vi "DAQ Loop.vi"(8 "error in":errorcluster, 10 "Queues":T1, 11 "Notifiers":T2) -> (0 "error out":errorcluster)   [LabVIEW 2015, in "DAQ.lvlib"]
uses:
  DAQ.lvlib
  support/Message Queue/Message Queue.lvlib
  TypeDefs/DAQ data.ctl
  <vilib>/ErrorRing/Error Ring.xnode
  PLC/PLC.lvlib
  support/Global names.vi
  <vilib>/Utility/error.llb/Error Cluster From Error Code.vi
  support/Message Queue/Message Cluster.ctl
  support/Notifiers/Notifiers.ctl
  support/Notifiers/Notifiers.lvlib
  support/Message Queue/All Message Queues.ctl
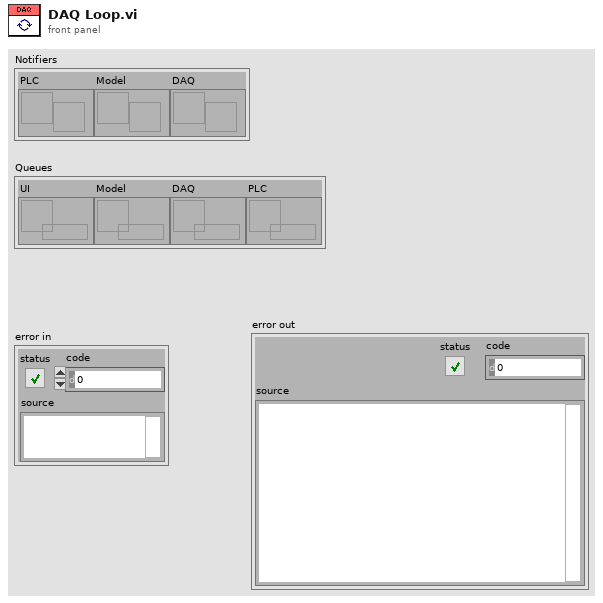
[diagram p1: front panel]
types:
  T1 = typedef "Message Queue.lvlib/All Message Queues.ctl" = cluster{"UI":refnum<queue>, "Model":refnum<queue>, "DAQ":refnum<queue>, "PLC":refnum<queue>}
  T2 = typedef "Notifiers.lvlib/Notifiers.ctl" = cluster{"PLC":refnum<notifier>, "Model":refnum<notifier>, "DAQ":refnum<notifier>}
  T3 = typedef "DAQ.lvlib/DAQ data.ctl" = cluster{"Power switch (DI)":cluster{"Channel":tag, "Data":bool}, "Dispose barrel (DI)":cluster{"Channel":tag, "Data":bool}, "Pump status (DO)":cluster{"Channel":tag, "Data":bool}, "Barrel position (AI)":cluster{"Channel":tag, "Data":dbl}}
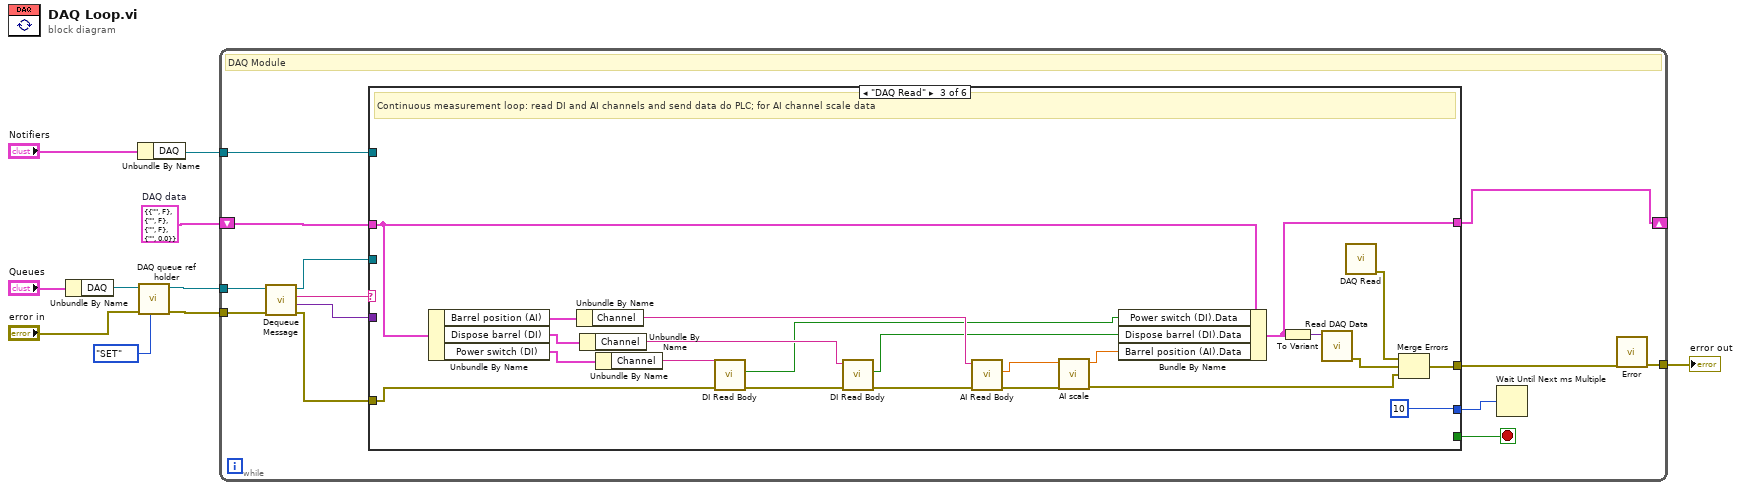
[diagram p0: block diagram]
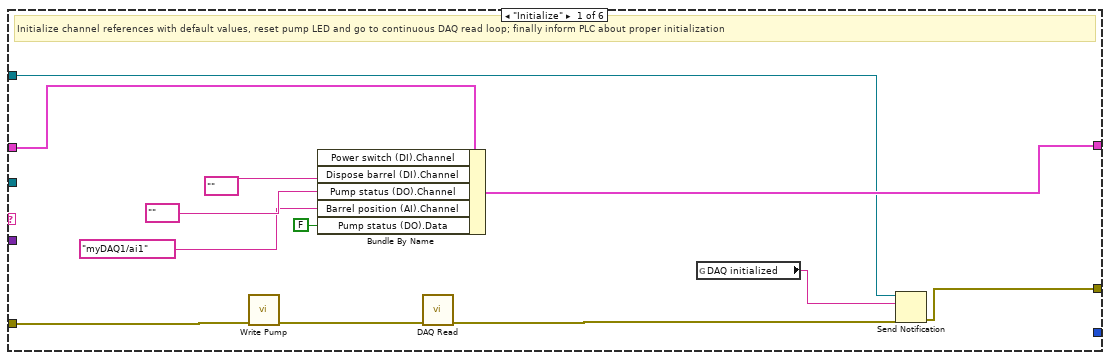
[diagram p2: hidden frame]
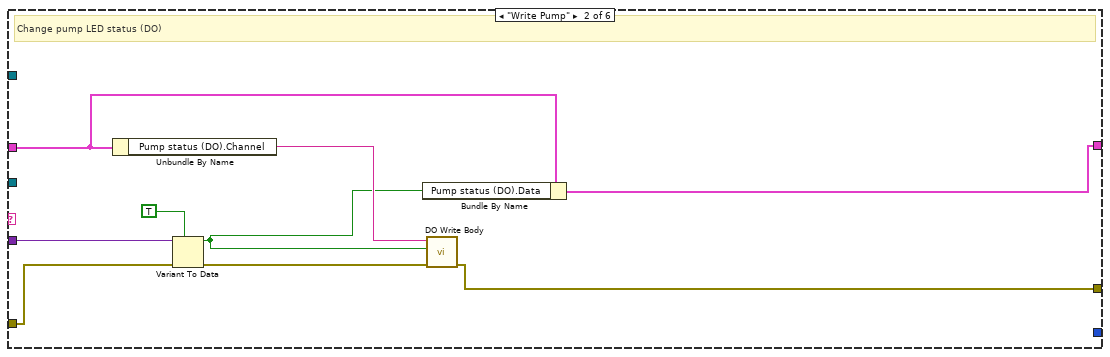
[diagram p3: hidden frame]
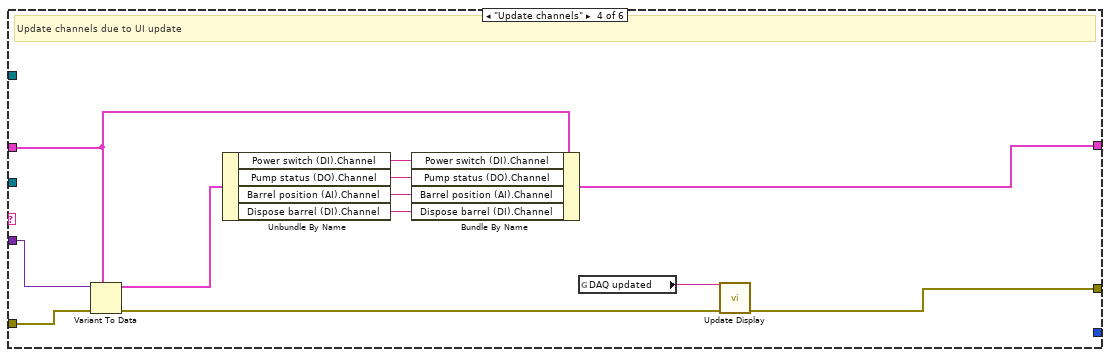
[diagram p4: hidden frame]
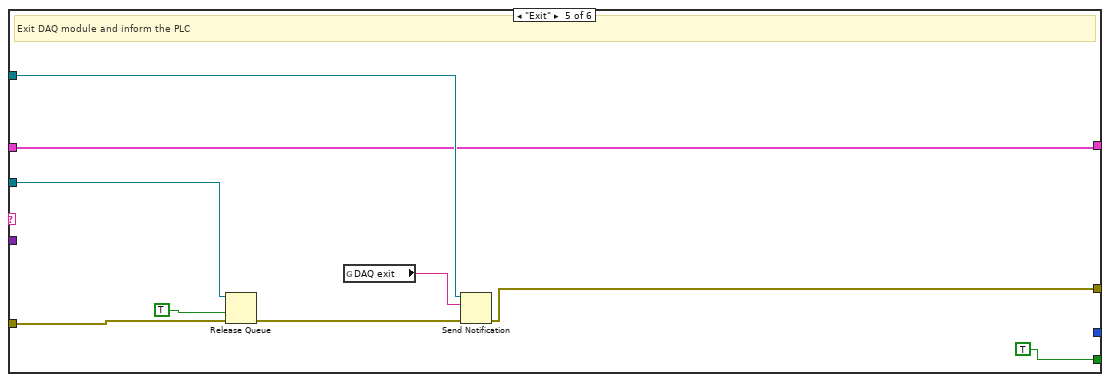
[diagram p5: hidden frame]
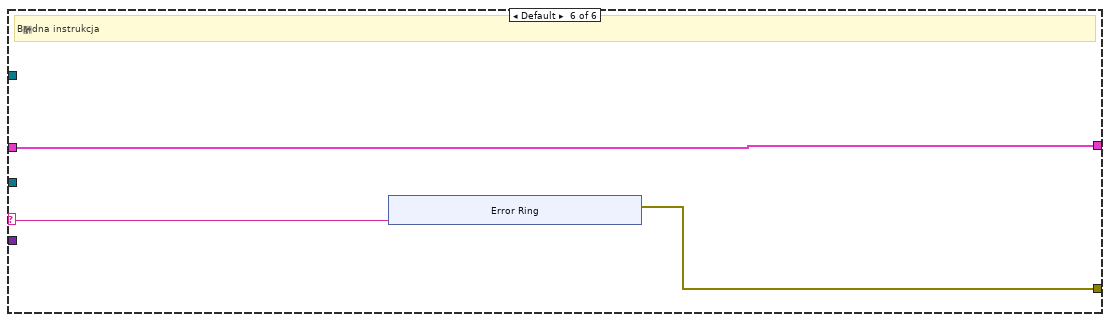
[diagram p6: hidden frame]
diagram:
  w10 = T3 {"Power switch (DI)"={"Channel"="", "Data"=FALSE}, "Dispose barrel (DI)"={"Channel"="", "Data"=FALSE}, "Pump status (DO)"={"Channel"="", "Data"=FALSE}, "Barrel position (AI)"={"Channel"="", "Data"=0.0}}  # DAQ data
  n1 = Unbundle By Name("Queues") -> ("DAQ"=w5:refnum<queue>)
  n2 = Unbundle By Name("Notifiers") -> ("DAQ"=w6:refnum<notifier>)
  n3 = call "DAQ queue ref holder.vi"("Action"=enum16{"GET", "SET"}."SET", "error in"="error in", "Message Queue In"=w5) -> ("error out"=w3:errorcluster, "Input Message Queue"=w4:refnum<queue>)  [unwired: 7 in]
  n4 = while {
    tunnel: w3 -> [w23]
    tunnel: w4 -> [w11]
    tunnel: w6 -> [w19]
    shift-right: [w18] -> _
    shift-left: w10 -> [w16]
    tunnel: [w14] -> w8
    stop <- w20 stop-if-true
    # "DAQ Module"
    n5 = call "Dequeue Message.vi"("error in (no error)"=w23, "Message Queue"=w11) -> ("error out"=w22:errorcluster, "Message Data"=w21:variant, "Message"=w12:string, "dup Message Queue"=w13:refnum<queue>)  [unwired: 6 in]
    n6 = case shown="\"DAQ Read\"" w12 {
      selector: w12 -> [_ _ _ _ _ w89]
      tunnel: w22 -> [w32 w44 w59 w77 w81 _]
      tunnel: [w35 w36 w57 w69 w80 w88] -> w15
      tunnel: w21 -> [_ w43 _ w78 _ _]
      tunnel: [_ _ _ _ TRUE _] -> w20
      tunnel: w13 -> [_ _ _ _ w87 _]
      tunnel: w19 -> [w30 _ _ _ w86 _]
      tunnel: w16 -> [w34 w40 w64 w76 w82 w90]
      tunnel: [w33 w42 w61 w71 w82 w90] -> w18
      tunnel: [_ _ u32 10 ("millisecond multiple") _ _ _] -> w17
      frame "Initialize" {
        # "Initialize channel references with default values, reset pump LED and go to continuous DAQ read loop; finally inform PLC about proper initialization"
        n7 = call "Write Pump.vi"("error in"=w32) -> ("error out"=w31:errorcluster)  [unwired: 10 in]
        n8 = Bundle By Name(cluster=w34, "Dispose barrel (DI).Channel"=tag "", "Pump status (DO).Channel"=tag "", "Barrel position (AI).Channel"=tag "myDAQ1/ai1", "Pump status (DO).Data"=FALSE) -> (w33:T3)  [unwired: 1 in]
        n9 = call "DAQ Read.vi"("error in"=w31) -> ("error out"=w29:errorcluster)  [unwired: 10 in]
        n10 = global read "Global names.vi" "DAQ initialized"() -> (w28:string)
        n11 = Send Notification(notification=w28, notifier=w30, error in (no error)=w29) -> (error out=w35:errorcluster)  [unwired: 1 out]
      }
      frame "Write Pump" {
        # "Change pump LED status (DO)"
        n12 = Unbundle By Name(w40) -> ("Pump status (DO).Channel"=w41:tag)
        n13 = Variant To Data(error in=w44, type=TRUE, Variant=w43) -> (data=w38:bool, error out=w37:errorcluster)
        n14 = Bundle By Name(cluster=w40, "Pump status (DO).Data"=w38) -> (w42:T3)
        n15 = call "DO Write Body.vi"("error in"=w37, "data"=w38, "Channel"=w41) -> ("error out"=w36:errorcluster)  [unwired: 6 in]
      }
      frame "DAQ Read" {
        # "Continuous measurement loop: read DI and AI channels and send data do PLC; for AI channel scale data"
        n16 = Unbundle By Name(w64) -> ("Barrel position (AI)"=w53:cluster{"Channel":tag, "Data":dbl}, "Dispose barrel (DI)"=w51:cluster{"Channel":tag, "Data":bool}, "Power switch (DI)"=w49:cluster{"Channel":tag, "Data":bool})
        n17 = Unbundle By Name(w53) -> ("Channel"=w52:tag)
        n18 = Unbundle By Name(w51) -> ("Channel"=w50:tag)
        n19 = Unbundle By Name(w49) -> ("Channel"=w48:tag)
        n20 = call "DI Read Body.vi"("error in"=w59, "Channel"=w48) -> ("error out"=w66:errorcluster, "data"=w47:bool)  [unwired: 6 in]
        n21 = call "DI Read Body.vi"("error in"=w66, "Channel"=w50) -> ("error out"=w65:errorcluster, "data"=w46:bool)  [unwired: 6 in]
        n22 = call "AI Read Body.vi"("error in"=w65, "Channel"=w52) -> ("error out"=w58:errorcluster, "data"=w54:dbl)  [unwired: 6 in]
        n23 = call "AI scale.vi"("error in"=w58, "Data in"=w54) -> ("error out"=w55:errorcluster, "Data out"=w63:dbl)  [unwired: 8 in]
        n24 = Bundle By Name(cluster=w64, "Power switch (DI).Data"=w47, "Dispose barrel (DI).Data"=w46, "Barrel position (AI).Data"=w63) -> (w61:T3)
        n25 = To Variant(anything=w61) -> (Variant=w60:variant)
        n26 = call "Read DAQ Data.vi"("Message Data"=w60) -> ("error out"=w56:errorcluster)  [unwired: 10 in]
        n27 = call "DAQ Read.vi"() -> ("error out"=w45:errorcluster)  [unwired: 11 in]
        n28 = Merge Errors(w45, w56, w55) -> (w57:errorcluster)
      }
      frame "Update channels" {
        # "Update channels due to UI update"
        n29 = Variant To Data(error in=w77, type=w76, Variant=w78) -> (data=w68:T3, error out=w70:errorcluster)
        n30 = Unbundle By Name(w68) -> ("Power switch (DI).Channel"=w75:tag, "Pump status (DO).Channel"=w74:tag, "Barrel position (AI).Channel"=w73:tag, "Dispose barrel (DI).Channel"=w72:tag)
        n31 = Bundle By Name(cluster=w76, "Power switch (DI).Channel"=w75, "Pump status (DO).Channel"=w74, "Barrel position (AI).Channel"=w73, "Dispose barrel (DI).Channel"=w72) -> (w71:T3)
        n32 = global read "Global names.vi" "DAQ updated"() -> (w67:string)
        n33 = call "Update Display.vi"("error in"=w70, "Message string"=w67) -> ("error out"=w69:errorcluster)  [unwired: 9 in]
      }
      frame "Exit" {
        # "Exit DAQ module and inform the PLC"
        n34 = Release Queue(queue=w87, force destroy? (F)=TRUE, error in (no error)=w81) -> (error out=w85:errorcluster)  [unwired: 2 out]
        n35 = global read "Global names.vi" "DAQ exit"() -> (w79:string)
        n36 = Send Notification(notification=w79, notifier=w86, error in (no error)=w85) -> (error out=w80:errorcluster)  [unwired: 1 out]
      }
      frame Default {
        # "B酬dna instrukcja"
        n37 = xnode "Error Ring"("parameter 0"=w89) -> ("error out"=w88:errorcluster)
      }
    }
    n38 = Wait Until Next ms Multiple(millisecond multiple=w17) -> ()  [unwired: 1 out]
    n39 = call "Error.vi"("error in"=w15) -> ("error out"=w14:errorcluster)  [unwired: 10 in]
  }
  "error out" <- w8
